vi "Gyro_Calibration.vi"(10 "Counts":dbl, 11 "GyroDevRef":T1={"DevStatus"={"status"=FALSE, "code"=0, "source"=""}, "Analog Module"=enum."Controller 1", "Analog Channel"=enum."AI 1", "Offset"=0.0, "Gain (VoltsPerDegree/Second)"=0.0}) -> (3 "Average":dbl)   [LabVIEW 2014]
uses:
  <vilib>/Rock Robotics/WPI/Gyro/WPI_GyroDevRef.ctl
  <vilib>/Rock Robotics/SystemInterfaces/Typedef/FPGA_TypedefAnalogModule.ctl
  <vilib>/Rock Robotics/SystemInterfaces/AI/FPGA_AIChannel.ctl
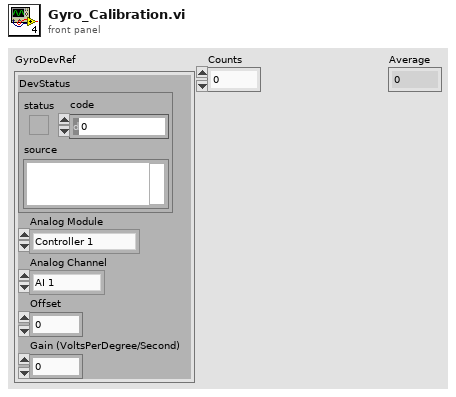
[diagram p1: front panel]
types:
  T1 = typedef "WPI_GyroDevRef.ctl" = cluster{"DevStatus":errorcluster, "Analog Module":T2, "Analog Channel":T3, "Offset":dbl, "Gain (VoltsPerDegree/Second)":dbl}
  T2 = typedef "FPGA_TypedefAnalogModule.ctl" = enum16{"Controller 1"}
  T3 = typedef "FPGA_AIChannel.ctl" = enum8{"AI 0", "AI 1", "AI 2", "AI 3", "AI MXP 0", "AI MXP 1", "AI MXP 2", "AI MXP 3", "Invalid"}
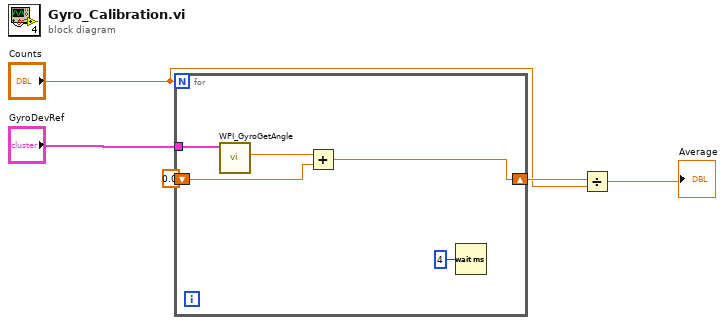
[diagram p0: block diagram]
diagram:
  n1 = for {
    N: "Counts" -> [_]
    shift-right: [w7] -> w3
    shift-left: 0.0 -> [w10]
    tunnel: "GyroDevRef" -> [w8]
    n2 = call <vilib>:"WPI_GyroGetAngle.vi"("GyroDevRef"=w8) -> ("Angle"=w6:dbl)  [unwired: 7 in, 3 out]
    n3 = Add(x=w6, y=w10) -> (x+y=w7:dbl)
    n4 = Wait (ms)(milliseconds to wait=u32 4) -> ()  [unwired: 1 out]
  }
  n5 = Divide(x=w3, y="Counts") -> (x/y=→"Average":dbl)
